vi "Inverse Kinematics Test.vi"() -> ()   [LabVIEW 2020]
uses:
  <vilib>/Analysis/Matrix/Datatypes/RealMatrix.ctl
  <vilib>/Analysis/Matrix/NI_Matrix.lvlib
panel:
  in  "stop":bool
  in  "Hide Components?":bool
  in  "dt":dbl
  in  "# Points":i32
  out "Expected Trajectory":cluster{dbl[], dbl[]}(graph)
  out "Forward Kinematics (Not tested)":T1
  in  "Angular Velocity":dbl(slide) scale=-180.0..180.0
  out "Arcade Inputs":picture
  out "Visualization":cluster{dbl[], dbl[]}[](graph)
  in  "Radii":T2={"LF"=[-2.0, 2.0], "LB"=[-2.0, -2.0], "RF"=[2.0, 2.0], "RB"=[2.0, -2.0]} {"RB" format="%.2f"; "RF" format="%.2f"; "LB" format="%.2f"; "LF" format="%.2f"}
  # "Front (1)"
  # "Left (-1)"
  # "Right (1)"
  # "Back (-1)"
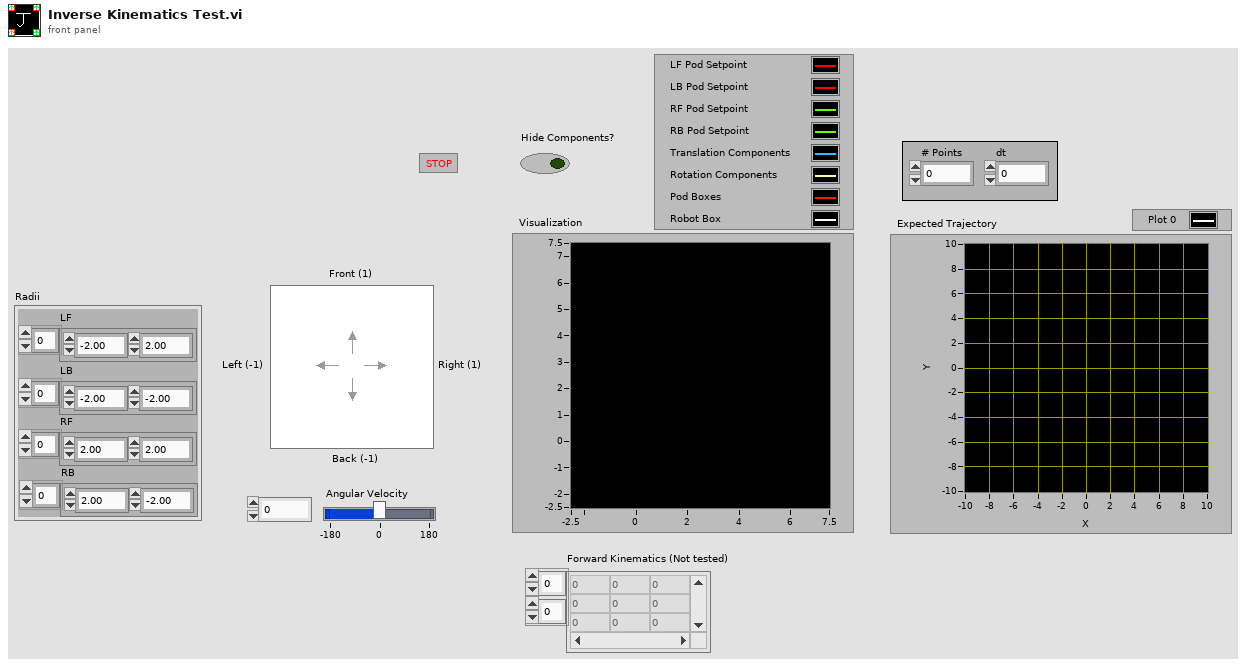
[diagram p1: front panel]
types:
  T1 = typedef "NI_Matrix.lvlib/RealMatrix.ctl" = dbl[][]
  T2 = cluster{"LF":dbl[], "LB":dbl[], "RF":dbl[], "RB":dbl[]}
  T3 = cluster{"Plot.Plot Color":u32, "Plot.Line Style":u8}
  T4 = typedef "LVMouseTypeDef.ctl" = cluster{"Mouse Position":cluster{"X":i32, "Y":i32}, "Mouse Modifiers":cluster{"Button Down":bool, "Shift Mod":bool, "Menu Mod":bool, "Option Mod":bool}}
  T5 = typedef "LVBoundsTypeDef.ctl" = cluster{"Width":u32, "Height":u32}
  T6 = cluster{"Theta":dbl, "Theta":dbl, "Theta":dbl, "Theta":dbl}
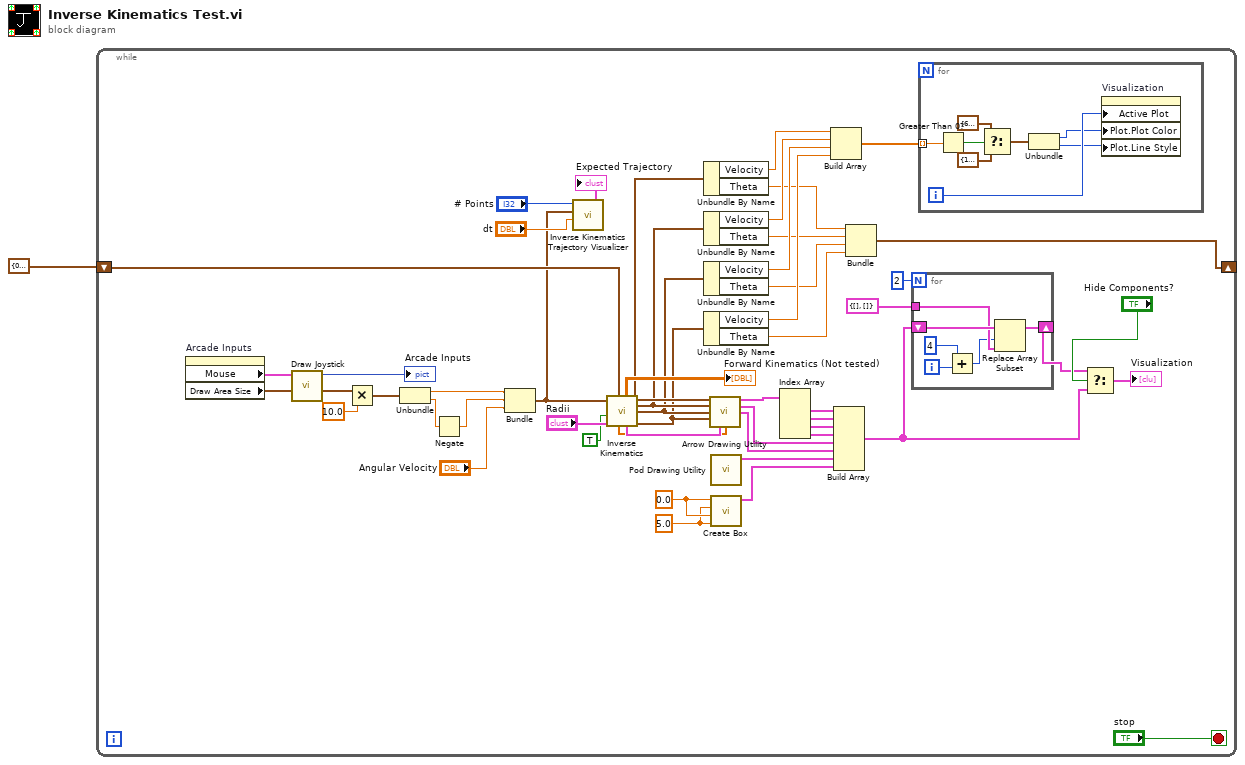
[diagram p0: block diagram]
diagram:
  n1 = while {
    shift-right: [w4] -> _
    shift-left: cluster{"LF":dbl, "LB":dbl, "RF":dbl, "RB":dbl} {"LF"=0.0, "LB"=0.0, "RF"=0.0, "RB"=0.0} ("Current Pod Steering") -> [w22]
    stop <- "stop" stop-if-true
    w51 = 5.0 ("Right")
    w52 = 0.0 ("Left")
    n2 = property on="Arcade Inputs" class="Pict"() -> ("Mouse"=w47:T4, "Draw Area Size"=w46:T5)  [unwired: 2 in, 2 out]
    n3 = call "Draw Joystick.vi"("Size"=w46, "Mouse"=w47) -> ("JS Coords"=w40:cluster{"X":dbl, "Y":dbl}, "Arcade Inputs"=→"Arcade Inputs":picture)  [unwired: 8 in]
    n4 = Multiply(x=w40, y=10.0 ("Angular Velocity")) -> (x*y=w39:cluster{"X":dbl, "Y":dbl})
    n5 = Unbundle(w39) -> ("X"=w12:dbl, "Y"=w45:dbl)
    n6 = Negate(x=w45) -> (-x=w11:dbl)
    n7 = Bundle("X"=w12, w11, "Angular Velocity"="Angular Velocity") -> (w9:cluster{"X":dbl, dbl, "Angular Velocity":dbl})  [unwired: 1 in]
    n8 = call "Inverse Kinematics Trajectory Visualizer.vi"("dt"="dt", "Target Velocity"=w9, "# Points"="# Points") -> ("Points"=→"Expected Trajectory":cluster{dbl[], dbl[]})  [unwired: 8 in]
    n9 = call "Inverse Kinematics.vi"("Current Pod Steering (deg)"=w22, "Radii (ft)"="Radii", "debug (F)"=TRUE, "Target Velocity (ft/s and deg/s)"=w9) -> ("RB Pod Setpoint (ft/s and deg/s)"=w18:cluster{"Velocity":dbl, "Theta":dbl}, "RF Pod Setpoint (ft/s and deg/s)"=w19:cluster{"Velocity":dbl, "Theta":dbl}, "LB Pod Setpoint (ft/s and deg/s)"=w20:cluster{"Velocity":dbl, "Theta":dbl}, "LF Pod Setpoint (ft/s and deg/s)"=w21:cluster{"Velocity":dbl, "Theta":dbl}, "cross products"=w37:T2, "A x B"=→"Forward Kinematics (Not tested)":T1, "translation"=w36:dbl[])  [unwired: 1 in]
    n10 = Unbundle By Name(w21) -> ("Velocity"=w17:dbl, "Theta"=w8:dbl)
    n11 = Unbundle By Name(w20) -> ("Velocity"=w16:dbl, "Theta"=w7:dbl)
    n12 = Unbundle By Name(w19) -> ("Velocity"=w15:dbl, "Theta"=w6:dbl)
    n13 = Unbundle By Name(w18) -> ("Velocity"=w14:dbl, "Theta"=w5:dbl)
    n14 = call "Arrow Drawing Utility.vi"("LF Pod Setpoint"=w21, "LB Pod Setpoint"=w20, "RF Pod Setpoint"=w19, "RB Pod Setpoint"=w18, "cross products"=w37, "Translation"=w36) -> ("Pod Vectors"=w31:cluster{dbl[], dbl[]}[], "Translation Vectors"=w35:cluster{dbl[], dbl[]}, "Rotation Vectors"=w34:cluster{dbl[], dbl[]})  [unwired: 7 in]
    n15 = call "Pod Drawing Utility.vi"() -> ("Cluster"=w49:cluster{dbl[], dbl[]})  [unwired: 11 in]
    n16 = call "Create Box.vi"("Top"=w51, "Bottom"=w52, "Right"=w51, "Left"=w52) -> ("Box"=w50:cluster{dbl[], dbl[]})  [unwired: 5 in, 2 out]
    n17 = Index Array(array=w31) -> (element #1=w30:cluster{dbl[], dbl[]}, element #2=w29:cluster{dbl[], dbl[]}, element #3=w28:cluster{dbl[], dbl[]}, element #4=w27:cluster{dbl[], dbl[]})  [unwired: 4 in]
    n18 = Build Array(w17, w16, w15, w14) -> (w13:dbl[])
    n19 = Build Array(w30, w29, w28, w27, w35, w34, w49, w50) -> (w26:cluster{dbl[], dbl[]}[])
    n20 = Bundle("Theta"=w8, "Theta"=w7, "Theta"=w6, "Theta"=w5) -> (w4:T6)  [unwired: 1 in]
    n21 = for {
      N: 2 -> [_]
      tunnel: cluster{dbl[], dbl[]} {[], []} ("new element/subarray") -> [w66]
      shift-right: [w65] -> w23
      shift-left: w26 -> [w67]
      i -> [w64]
      n22 = Add(x=4, y=w64) -> (x+y=w62:i32)
      n23 = Replace Array Subset(array=w67, new element=w66, index=w62) -> (w65:cluster{dbl[], dbl[]}[])
    }
    n24 = for {
      tunnel: w13 -> [w60] mode=indexing
      i -> [w61]
      n25 = Greater Than 0?(x=w60) -> (x > 0?=w59:bool)
      n26 = Select(t=T3 {"Plot.Plot Color"=6618880, "Plot.Line Style"=0}, s=w59, f=T3 {"Plot.Plot Color"=16711680, "Plot.Line Style"=2}) -> (s? t:f=w56:T3)
      n27 = Unbundle(w56) -> ("Plot.Plot Color"=w55:u32, "Plot.Line Style"=w54:u8)
      n28 = property on="Visualization" class="XYGraph (strict)"("Active Plot"=w61, "Plot.Plot Color"=w55, "Plot.Line Style"=w54) -> ()  [unwired: 2 in, 2 out]
    }
    n29 = Select(t=w23, s="Hide Components?", f=w26) -> (s? t:f=→"Visualization":cluster{dbl[], dbl[]}[])
  }
